vi "DmgrOpen.vi"(8 "Error In":errorcluster, 11 "Device Name":string) -> (0 "Error Out":errorcluster, 3 "HIF":u32)   [LabVIEW 2011, in "LVH-Adept.lvlib" / "DMGR.lvlib"]
uses:
  DMGR.lvlib
  Private/Type Defs/Error.ctl
  Resources/dmgr.dll
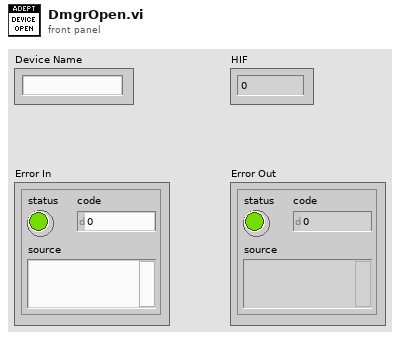
[diagram p1: front panel]
types:
  T1 = typedef "LVH-Adept.lvlib/DMGR.lvlib/Error.ctl" = enum16{"Unknown Error", "Device Enumeration", "Device Handle", "Device Info", "Device Open"}
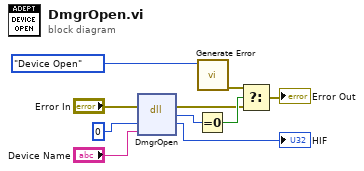
[diagram p0: block diagram]
diagram:
  n1 = dll-call lib="C:/github/labviewhacker/LVH-Adept/LabVIEW/vi.lib/LabVIEW Hacker/Adept/Private/Resources/dmgr.dll" fn="DmgrOpen"(error in="Error In", "phif"=u32 0, "szSel"="Device Name") -> (error out=w3:errorcluster, "Success"=w8:u32, "phif"=→"HIF":u32)  [unwired: 3 in, 1 out]
  n2 = Equal To 0?(x=w8) -> (x = 0?=w6:bool)
  n3 = call "Generate Error.vi"("Error Type"=Error."Device Open") -> ("Error Out"=w4:errorcluster)  [unwired: 10 in]
  n4 = Select(t=w4, s=w6, f=w3) -> (s? t:f=→"Error Out":errorcluster)
